vi "test Read Default Tag Distance Array.vi"(8 "error in (no error)":errorcluster, 11 "TestCase in":refnum<class "AnchorTests.lvclass">) -> (0 "error out":errorcluster, 3 "TestCase out":refnum<class "AnchorTests.lvclass">)   [LabVIEW 2014, in "AnchorTests.lvclass"]
uses:
  AnchorTests.lvclass
  SPLAT/Anchor/Anchor.lvclass
  <vilib>/addons/_JKI Toolkits/VI Tester/TestCase.llb/TestCase.lvclass
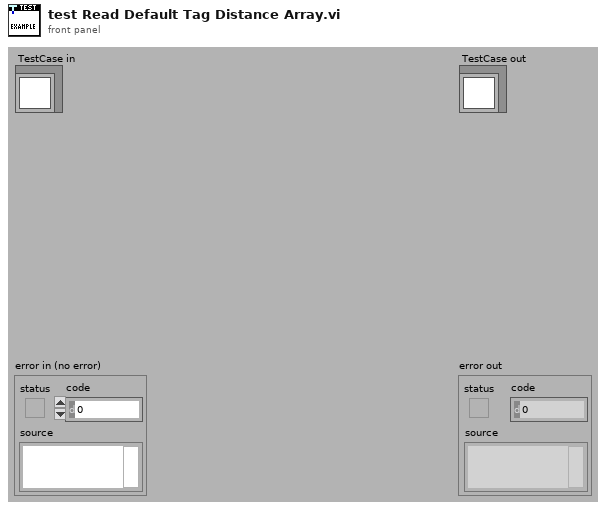
[diagram p1: front panel]
types:
  T1 = cluster{"Tag.lvclass":refnum<class "Tag.lvclass">, "Distance":dbl}[]
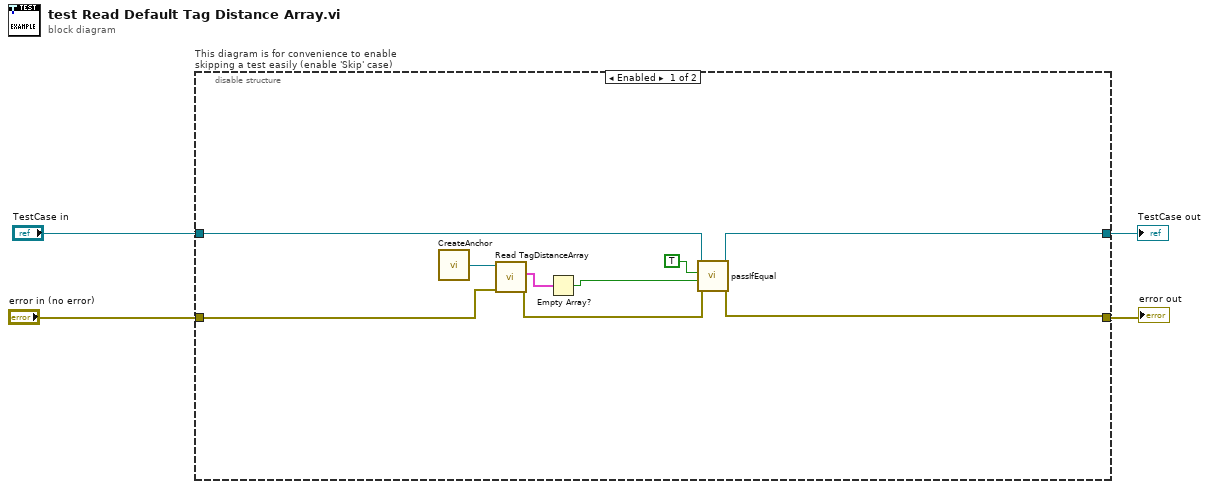
[diagram p0: block diagram]
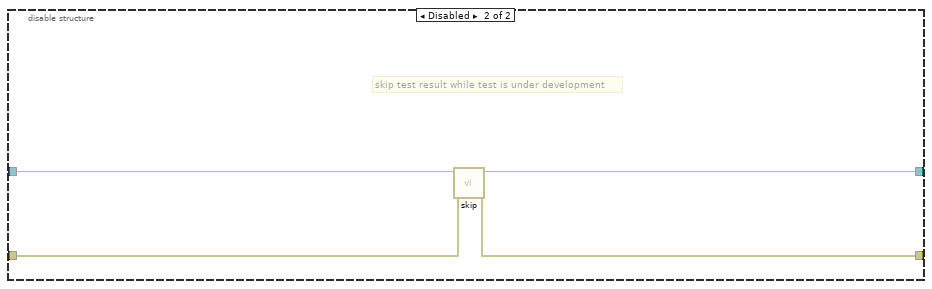
[diagram p2: hidden frame]
diagram:
  n1 = disable-structure "This diagram is for convenience to enable skipping a test easily (enable 'Skip' case)" shown="Enabled" {
    disable-tunnel: "TestCase in" -> [w13 w17]
    disable-tunnel: [w12 w15] -> w1
    disable-tunnel: [w11 w16] -> w3
    disable-tunnel: "error in (no error)" -> [w9 w14]
    frame Enabled {
      n2 = call "CreateAnchor.vi"() -> ("Anchor Out"=w10:refnum<class "Anchor.lvclass">)  [unwired: 3 in]
      n3 = call-dynamic "Read TagDistanceArray.vi"("error in (no error)"=w9, "Anchor in"=w10) -> ("error out"=w8:errorcluster, "TagDistanceArray"=w7:T1)  [unwired: 7 in, 1 out]
      n4 = Empty Array?(array=w7) -> (empty?=w6:bool)
      n5 = call-dynamic "passIfEqual.vi"("error in (no error)"=w8, "y"=w6, "x"=TRUE, "TestCase in"=w13) -> ("error out"=w11:errorcluster, "TestCase out"=w12:refnum<class "AnchorTests.lvclass">)  [unwired: 6 in]
    }
    frame Disabled {
      # "skip test result while test is under development"
      n6 = call <vilib>:"skip.vi"("error in (no error)"=w14, "TestCase in"=w17) -> ("error out"=w16:errorcluster, "TestCase out"=w15:refnum<class "AnchorTests.lvclass">)  [unwired: 8 in]
    }
  }
  "error out" <- w3
  "TestCase out" <- w1
